vi "On Stop.vi"(6 "Diagnostics Queue":refnum<queue>, 7 "Host Resources":T1, 8 "error in (no error)":errorcluster, 11 "Hardware Configuration in":T4) -> (0 "error out":errorcluster, 3 "Hardware Configuration out":T4)   [LabVIEW 2021, in "Acquisition.lvlib"]
doc: "Stop the acquisition."
uses:
  Acquisition.lvlib
  Hardware Configuration.ctl
  Channel Settings.ctl
  IO Device.ctl
  Sensor Type.ctl
  Interval Timer/Repeat Interval.ctl
  Interval Timer/Interval Length.ctl
  Interval Timer/Interval Token.ctl
  IO Context.ctl
  IO API.ctl
  support/Message Queue/Message Cluster.ctl
  Host Resources.ctl
  Host Software Package.ctl
  Host IO Resource.ctl
  Interval Timer/Interval Timer.lvlib
  support/Message Queue/Message Queue.lvlib
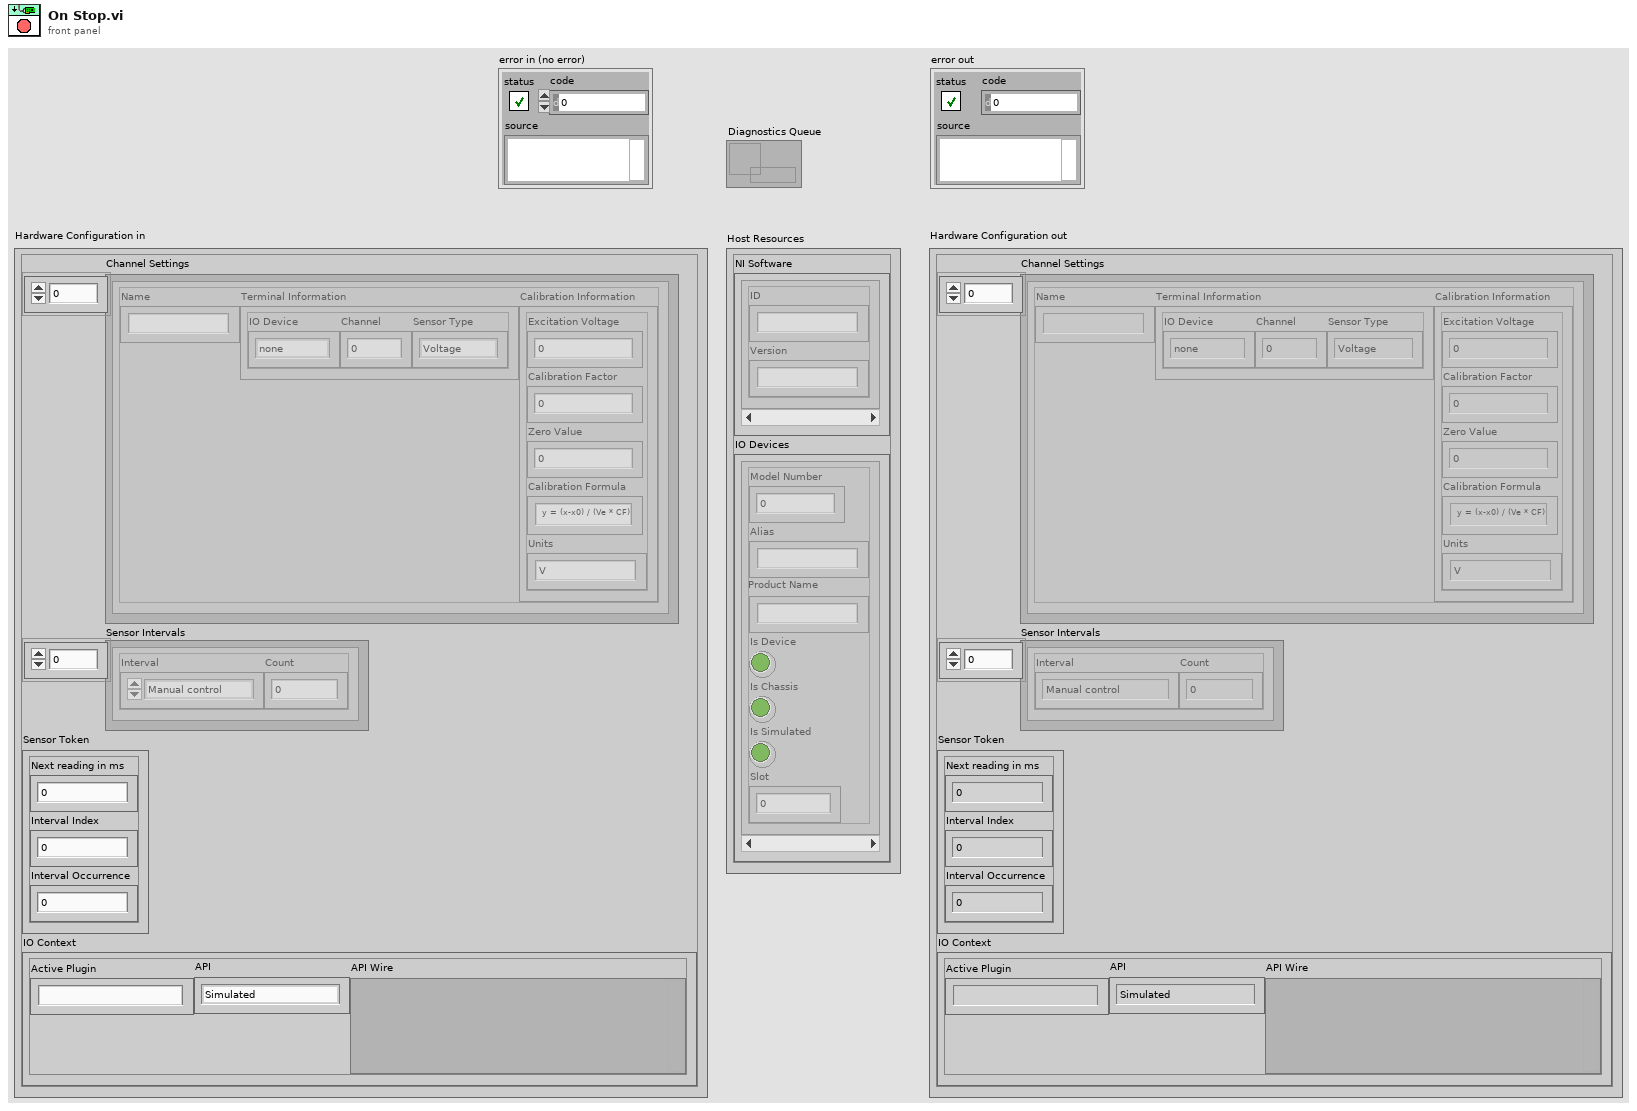
[diagram p1: front panel]
types:
  T1 = typedef "Acquisition.lvlib/Host Resources.ctl" = cluster{"NI Software":T2[], "IO Devices":T3[]}
  T2 = typedef "Acquisition.lvlib/Host Software Package.ctl" = cluster{"ID":string, "Version":string}
  T3 = typedef "Acquisition.lvlib/Host IO Resource.ctl" = cluster{"Model Number":u32, "Alias":string, "Product Name":string, "Is Device":bool, "Is Chassis":bool, "Is Simulated":bool, "Slot":i32}
  T4 = typedef "Acquisition.lvlib/Hardware Configuration.ctl" = cluster{"Channel Settings":T5[], "Sensor Intervals":T8[], "Sensor Token":T10, "IO Context":T11}
  T5 = typedef "Acquisition.lvlib/Channel Settings.ctl" = cluster{"Name":string, "Terminal Information":cluster{"IO Device":T6, "Channel":i32, "Sensor Type":T7}, "Calibration Information":cluster{"Excitation Voltage":dbl, "Calibration Factor":dbl, "Zero Value":dbl, "Calibration Formula":string, "Units":string}}
  T6 = typedef "Acquisition.lvlib/IO Device.ctl" = enum16{"none", "9219", "9401"}
  T7 = typedef "Acquisition.lvlib/Sensor Type.ctl" = enum16{"Voltage", "Load", "Pressure", "Encoder"}
  T8 = typedef "Interval Timer.lvlib/Repeat Interval.ctl" = cluster{"Interval":T9, "Count":i32}
  T9 = typedef "Interval Timer.lvlib/Interval Length.ctl" = enum16{"Manual control", "1 second", "10 seconds", "30 seconds", "60 seconds", "600 seconds", "1200 seconds", "3600 seconds"}
  T10 = typedef "Interval Timer.lvlib/Interval Token.ctl" = cluster{"Next reading in ms":u32, "Interval Index":i32, "Interval Occurrence":i32}
  T11 = typedef "Acquisition.lvlib/IO Context.ctl" = cluster{"Active Plugin":string, "API":T12, "API Wire":variant}
  T12 = typedef "Acquisition.lvlib/IO API.ctl" = enum16{"Simulated", "DAQmx"}
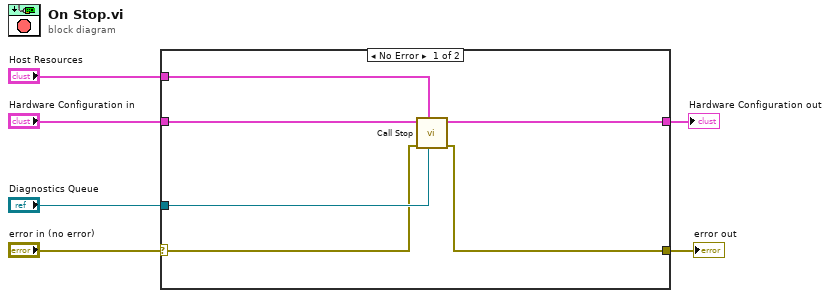
[diagram p0: block diagram]
diagram:
  n1 = case shown="No Error" "error in (no error)" {
    selector: "error in (no error)" -> [w11 w14]
    tunnel: [w7 w14] -> w5
    tunnel: "Hardware Configuration in" -> [w9 w13]
    tunnel: [w8 w13] -> w3
    tunnel: "Diagnostics Queue" -> [w12 _]
    tunnel: "Host Resources" -> [w10 _]
    frame No Error {
      n2 = call "Call Stop.vi"("Diagnostics Queue in"=w12, "Host Resources"=w10, "error in (no error)"=w11, "Hardware Configuration in"=w9) -> ("error out"=w7:errorcluster, "Hardware Configuration out"=w8:T4)  [unwired: 6 in]
    }
    frame Error {
    }
  }
  "error out" <- w5
  "Hardware Configuration out" <- w3
